vi "Readable String.vi"(11 "LowLimit Condition in":refnum<class "LowLimit Condition.lvclass">) -> (2 "String":string)   [LabVIEW 2020, in "VolatusSeq.lvlib" / "LowLimit Condition.lvclass"]
uses:
  LowLimit Condition.lvclass
  LowLimit Condition.lvclass/LowLimit Condition.ctl
  lv-vecto/Vecto/Channel DBL/Channel DBL.lvclass
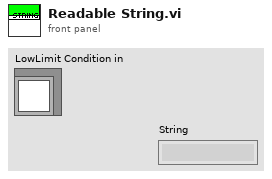
[diagram p1: front panel]
types:
  T1 = typedef "VectoConfig.lvlib/Channel Info.ctl" = cluster{"Name":string, "Group":string, "Owning Node":string, "Owning Task":string, "Resource":string}
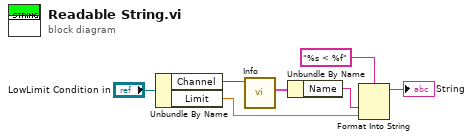
[diagram p0: block diagram]
diagram:
  n1 = Unbundle By Name("LowLimit Condition in") -> ("Channel"=w6:refnum<class "Channel DBL.lvclass">, "Limit"=w3:dbl)
  n2 = call "Info.vi"("Channel in"=w6) -> ("Info"=w5:T1)  [unwired: 8 in, 2 out]
  n3 = Unbundle By Name(w5) -> ("Name"=w4:string)
  n4 = Format Into String(format string="%s < %f", w4, w3) -> (resulting string=→"String":string)  [unwired: 2 in, 1 out]
